vi "SiosIfmMaxDeviceCount.vi"() -> (0 "maximum allowed devices":i32)   [LabVIEW 2009]
uses:
  siosifm.dll
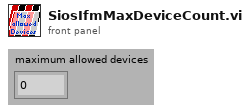
[diagram p1: front panel]
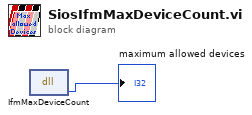
[diagram p0: block diagram]
diagram:
  n1 = dll-call lib="C:/WORK/Artem/RE-10/SIOS_IfmDLL/siosifm.dll" fn="IfmMaxDeviceCount"() -> ("IfmMaxDeviceCount"=→"maximum allowed devices":i32)  [unwired: 3 in, 2 out]
